vi "Compute Cache.vi"(8 "error in (no error)":errorcluster, 11 "httpResponse in":refnum<class "httpResponse.lvclass">) -> (0 "error out":errorcluster, 3 "httpResponse out":refnum<class "httpResponse.lvclass">)   [LabVIEW 2020, in "httpClient.lvlib" / "httpResponse.lvclass"]
uses:
  httpResponse.lvclass
  httpResponse.lvclass/httpResponse.ctl
  httpHeaders/httpHeaders.lvclass
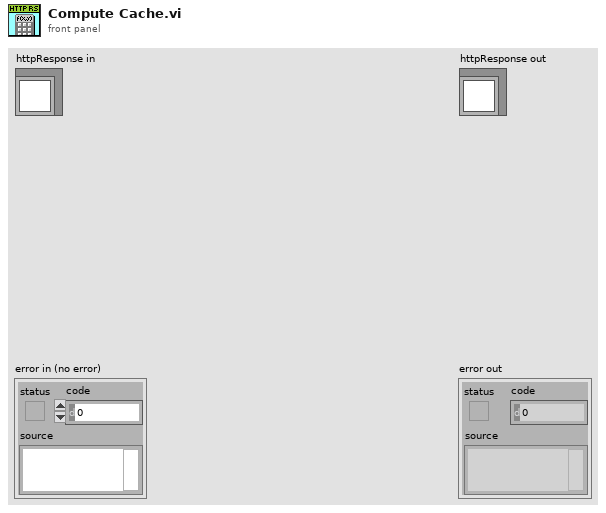
[diagram p1: front panel]
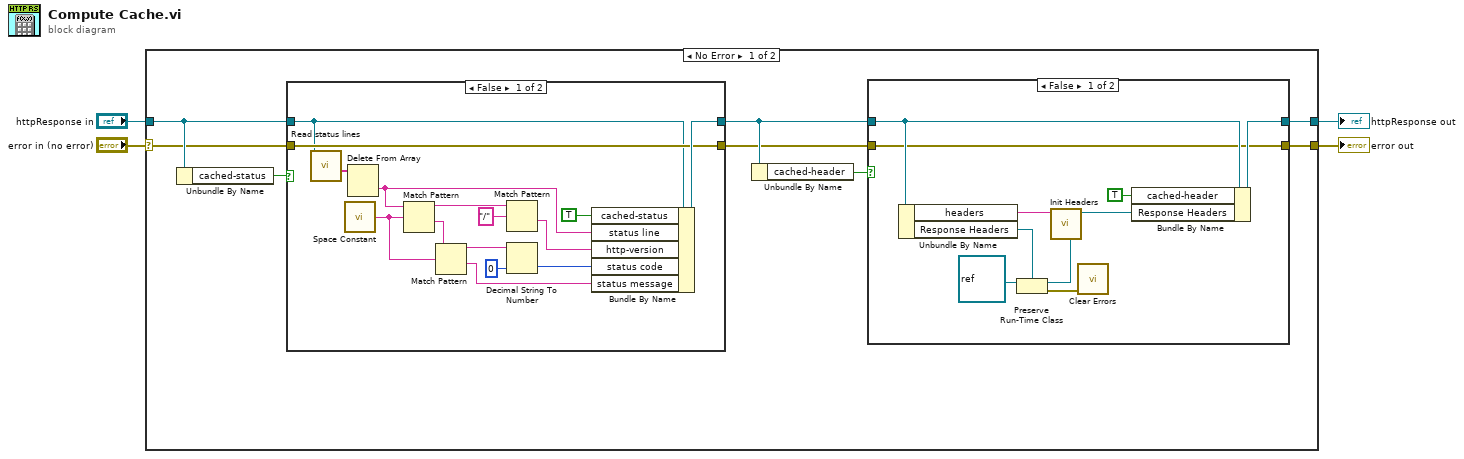
[diagram p0: block diagram]
diagram:
  n1 = case shown="No Error" "error in (no error)" {
    selector: "error in (no error)" -> [w10 w43]
    tunnel: [w7 w43] -> w3
    tunnel: [w8 w42] -> w1
    tunnel: "httpResponse in" -> [w12 w42]
    frame No Error {
      n2 = Unbundle By Name(w12) -> ("cached-status"=w11:bool)
      n3 = case shown="False" w11 {
        tunnel: [w27 w29] -> w9
        tunnel: w12 -> [w15 w29]
        tunnel: [w26 w28] -> w6
        tunnel: w10 -> [w26 w28]
        frame False {
          n4 = call "Read status lines.vi"("httpResponse in"=w15) -> ("status chain"=w14:string[])  [unwired: 8 in, 2 out]
          n5 = call <vilib>:"Space Constant.vi"() -> ("String"=w23:string)
          n6 = Delete From Array(array=w14) -> (deleted portion=w13:string)  [unwired: 2 in, 1 out]
          n7 = Match Pattern(string=w13, regular expression=w23) -> (before substring=w19:string, after substring=w20:string)  [unwired: 1 in, 2 out]
          n8 = Match Pattern(string=w20, regular expression=w23) -> (before substring=w22:string, after substring=w16:string)  [unwired: 1 in, 2 out]
          n9 = Match Pattern(string=w19, regular expression="/") -> (after substring=w18:string)  [unwired: 1 in, 3 out]
          n10 = Decimal String To Number(string=w22, default (0L)=u16 0 ("default (0 I32)")) -> (number=w17:u16)  [unwired: 1 in, 1 out]
          n11 = Bundle By Name(cluster=w15, "cached-status"=TRUE ("cached"), "status line"=w13, "http-version"=w18, "status code"=w17, "status message"=w16) -> (w27:refnum<class "httpResponse.lvclass">)
        }
        frame True {
        }
      }
      n12 = Unbundle By Name(w9) -> ("cached-header"=w5:bool)
      n13 = case shown="False" w5 {
        tunnel: w9 -> [w32 w40]
        tunnel: [w39 w40] -> w8
        tunnel: [w31 w41] -> w7
        tunnel: w6 -> [w31 w41]
        frame False {
          n14 = Unbundle By Name(w32) -> ("headers"=w36:string, "Response Headers"=w37:refnum<class "httpHeaders.lvclass">)
          n15 = Preserve Run-Time Class(object in=refnum<class> refnum ("LabVIEW Object"), 2:w37) -> (object out=w34:refnum<class "httpHeaders.lvclass">, error out=w33:errorcluster)  [unwired: 1 in]
          n16 = call "Init Headers.vi"("httpHeaders in"=w34, "http-header (unparsed)"=w36) -> ("httpHeaders out"=w30:refnum<class "httpHeaders.lvclass">)  [unwired: 9 in]
          n17 = call <vilib>:"Clear Errors.vi"("error in (no error)"=w33) -> ()  [unwired: 5 in, 2 out]
          n18 = Bundle By Name(cluster=w32, "cached-header"=TRUE, "Response Headers"=w30) -> (w39:refnum<class "httpResponse.lvclass">)
        }
        frame True {
        }
      }
    }
    frame Error {
    }
  }
  "error out" <- w3
  "httpResponse out" <- w1
